vi "sincos.vi"(11 "x (pi)":fxp<+/-,16,1> format="%#_20g") -> (2 "cos(x)":fxp<+/-,16,2>, 3 "sin(x)":fxp<+/-,16,2>)   [LabVIEW 2015]
doc: "Computes the sine and cosine of x. x is assumed to be in pi radians."
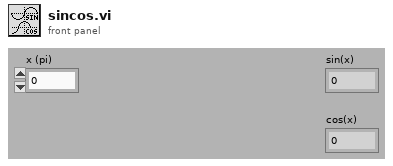
[diagram p1: front panel]
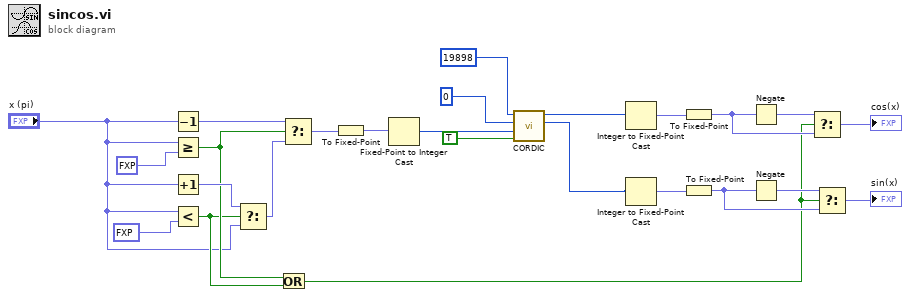
[diagram p0: block diagram]
diagram:
  n1 = Decrement(x="x (pi)") -> (x-1=w23:fxp<+/-,16,1>)
  n2 = Greater Or Equal?(x="x (pi)", y=fxp<+/-,16,1> 0.5) -> (x >= y?=w19:bool)
  n3 = Increment(x="x (pi)") -> (x+1=w22:fxp<+/-,16,1>)
  n4 = Less?(x="x (pi)", y=fxp<+/-,16,1> -0.5) -> (x < y?=w18:bool)
  n5 = Select(t=w22, s=w18, f="x (pi)") -> (s? t:f=w21:fxp<+/-,16,1>)
  n6 = Or(x=w19, y=w18) -> (x .or. y?=w7:bool)
  n7 = Select(t=w23, s=w19, f=w21) -> (s? t:f=w15:fxp<+/-,16,1>)
  n8 = To Fixed-Point(number=w15) -> (fixed-point=w6:fxp<+/-,17,1>)  [unwired: 1 in]
  n9 = Fixed-Point to Integer Cast(1:w6) -> (0:w5:i32)
  n10 = call "CORDIC.vi"("rotate"=TRUE ("Rotate"), "z"=w5, "y"=0 ("17.2(0)"), "x"=19898 ("17.2(0.6073)")) -> ("y'"=w3:i32, "x'"=w4:i32)  [unwired: 5 in, 1 out]
  n11 = Integer to Fixed-Point Cast(integer=w4) -> (fixed-point=w1:fxp<+/-,17,2>)  [unwired: 1 in]
  n12 = Integer to Fixed-Point Cast(integer=w3) -> (fixed-point=w2:fxp<+/-,17,2>)  [unwired: 1 in]
  n13 = To Fixed-Point(number=w1) -> (fixed-point=w10:fxp<+/-,16,2>)  [unwired: 1 in]
  n14 = To Fixed-Point(number=w2) -> (fixed-point=w11:fxp<+/-,16,2>)  [unwired: 1 in]
  n15 = Negate(x=w10) -> (-x=w12:fxp<+/-,16,2>)
  n16 = Negate(x=w11) -> (-x=w13:fxp<+/-,16,2>)
  n17 = Select(t=w12, s=w7, f=w10) -> (s? t:f=→"cos(x)":fxp<+/-,16,2>)
  n18 = Select(t=w13, s=w7, f=w11) -> (s? t:f=→"sin(x)":fxp<+/-,16,2>)
